vi "AlliGator Image Pre-processing.vi"(5 "Image Pre-Processing Parameters":T1 {"Hot Pixel Removal"."Percentile" min=0 max=100}, 6 "Data":sgl[][](array[numeric]), 7 "Buffer Image available?":bool, 8 "error in (no error)":errorcluster, 9 "Current Gate":i32, 10 "Refnum in":T6, 11 "Dataset Images in":T7) -> (0 "error out":errorcluster, 1 "Current Gate (dup)":i32, 2 "# Replacements":i32, 3 "Dataset Images out":T7, 4 "Image Resolution":cluster{"X Resolution":i32, "Y Resolution":i32})   [LabVIEW 2021, in "AlliGator Files.lvlib"]
doc: "Applies selected preprocessing steps to a gate image."
uses:
  AlliGator Files.lvlib
  AlliGator Gate Image Set.ctl
  <vilib>/vision/Image Controls.llb/IMAQ Image.ctl
  AlliGator Image Pre-processing Parameters.ctl
  Arrays/Kernel Type.ctl
  Arrays/Smoothing Algorithm.ctl
  SwissSPAD/SwissSPAD Live_Image Display Options.ctl
  AlliGator Image Pre-processing Step.ctl
  AlliGator Settings List.ctl
  de9ca15b-1b35-494c-9863-d7c52523ff08.vi
  a9c29a31-92f7-4b3b-9283-b1d6627186df.vi
  Arrays/n x n Kernel Convolution (SGL).vi
  Arrays/n x n Smoothen Array (SGL) v3.vi
  Arrays/n x n Kernel Convolution (SGL).vi/d0ebc029-cbaa-4c82-a58c-923c59c440da.vi
  Arrays/n x n Kernel Convolution (SGL).vi/b80d5e79-a0c8-46e2-aba9-3d60e0093a16.vi
  <vilib>/Analysis/2dsp.llb/Convolution.vi
  <vilib>/Analysis/2dsp.llb/2D Convolution (DBL).vi
  Arrays/Truncate Kernel.vi
  Arrays/Replace NaN by 0 (2D SGL).vi
  Arrays/n x n Smoothen Array (SGL) v3.vi/d0ebc029-cbaa-4c82-a58c-923c59c440da.vi
  Arrays/n x n Smoothen Array (SGL) v3.vi/b80d5e79-a0c8-46e2-aba9-3d60e0093a16.vi
  Arrays/Replace NaN by 0 (2D SGL).vi/df975b44-f6c5-4554-af30-980613d33749.vi
  Variant/Variant to Data/Variant to Boolean.vi
  Time/High Resolution Timing.vi
  Arrays/Compute n x n Kernel (SGL).vi
  <vilib>/Utility/error.llb/Simple Error Handler.vi
  Arrays/Arrays.lvlib
  AlliGator Settings.lvlib
  Variant/Variant to Data/Variant to Data.lvlib
  AlliGator Internal Variables.lvlib
  SwissSPAD/SwissSPAD Live.lvlib
panel:
  # "see the AlliGator License on the block diagram (Ctrl+E or Window:Show Block Diagram)"
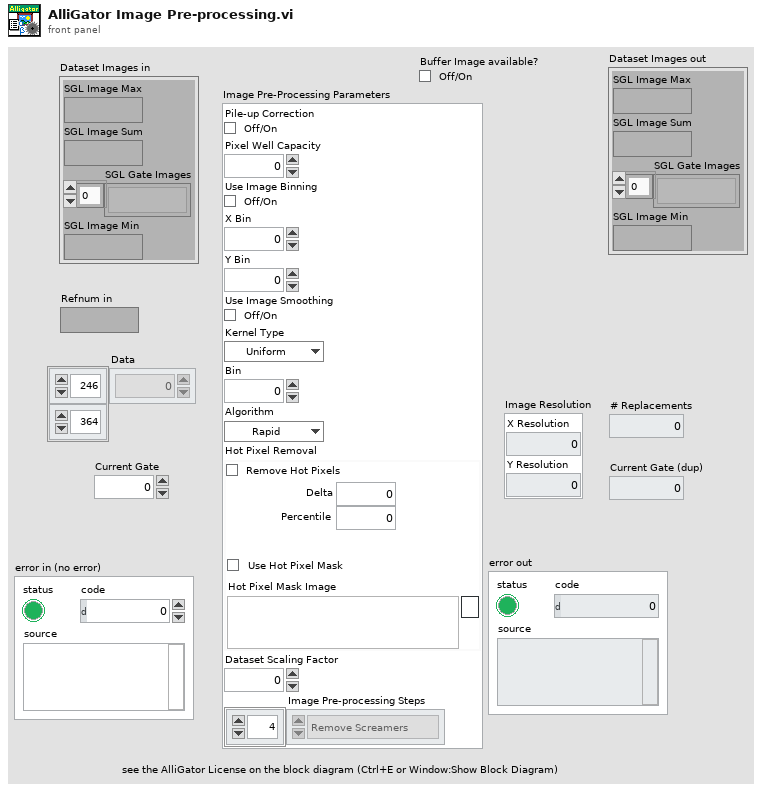
[diagram p1: front panel]
types:
  T1 = typedef "AlliGator Files.lvlib/AlliGator Image Pre-processing Parameters.ctl" = cluster{"Pile-up Correction":bool, "Pixel Well Capacity":u32, "Use Image Binning":bool, "X Bin":i32, "Y Bin":i32, "Use Image Smoothing":bool, "Kernel Type":T2, "Bin":i32, "Algorithm":T3, "Hot Pixel Removal":T4, "Dataset Scaling Factor":dbl, "Image Pre-processing Steps":T5[]}
  T2 = typedef "Arrays.lvlib/Kernel Type.ctl" = enum16{"Uniform", "Bilinear", "Gaussian"}
  T3 = typedef "Arrays.lvlib/Smoothing Algorithm.ctl" = enum16{"Rapid", "Thorough"}
  T4 = typedef "SwissSPAD Live.lvlib/SwissSPAD Live_Image Display Options.ctl" = cluster{"Remove Screamers":bool, "Delta":sgl, "Equalize Histogram":bool, "Percentile":sgl, "Hot Pixel Mask Image":path, "Use Hot Pixel Mask":bool}
  T5 = typedef "AlliGator Files.lvlib/AlliGator Image Pre-processing Step.ctl" = enum16{"Remove Screamers", "Pile-up Correction", "Binning", "Smoothing", "Rescaling", "Dead Left Column Correction"}
  T6 = typedef "IMAQ Image.ctl" = refnum<image>
  T7 = typedef "AlliGator Internal Variables.lvlib/AlliGator Gate Image Set.ctl" = cluster{"SGL Image Max":T6, "SGL Image Sum":T6, "SGL Gate Images":T6[], "SGL Image Min":T6}
  T8 = typedef "AlliGator Settings.lvlib/AlliGator Settings List.ctl" = enum16{"GUI:Visible Settings Tab", "GUI:Last Run Version", "Source Image:Use Image Histogram for Contrast", "Source Image:Low Count Pixels Rejection Options", "Source Image:High Count Pixels Rejection Options", "Source Image:Use Image Brightness", "Source Image:Blend Overlay with Image Background", "Source Image:Use Fixed ROI Diameter", "Source Image:ROI Diameter", "Source Image:ROI Center Color", "Source Image:Peak Threshold", "Source Image:Intensity Threshold", "Source Image:Image Binning Options", "Source Image:Image Smoothing Options", "Source Image:Image Histogram Active", "Source Image:Invert Binary Mask", "Source Image:Hot Pixel Removal", "Source Image:Overlay Analyzed ROI Center", "Source Image:Auto-Adjust Contrast", "Source Image:Histogram Lower Percentile", "Source Image:Histogram Upper Percentile", "Source Image:Save Source Image", "Source Image:Scale Bar Options", "Source Image:Image Resolution (Pixel Size)", "Source Image:Flatfield Correction", "Source Image:Show Dead Left Columns Correction", "Source Image:Dead Left Columns Correction", "Source Image:Image Pre-Processing Operations Order", "Data Information:Gate Width", "Data Information:Nanotime Gate Separation", "Data Information:Macrotime Gate Separation", "Data Information:Gate Step", "Data Information:# Gates", "Data Information:Gate Image Exposure", "Data Information:Gate Image Integration", "Data Information:Gates to Skip", "Data Information:Gates to Keep", "Data Information:Define Gates to", "Data Information:Channel Name", "Data Information:Available Channel Names", "Data Information:Channel Arithmetic", "Data Information:Background File Subtraction", "Data Information:Background File", "Data Information:Background Scaling Factor", "Data Information:Background Pile-up Correction", "Data Information:Background Pixel Well Capacity", "Data Information:Laser Period", "Data Information:SYNC Period", "Data Information:Pile-up Correction", "Data Information:Pixel Well Capacity", "Data Information:Dataset Scaling Factor", "Fluorescence Decay_Decay Pre-Processing:Reverse Gates", "Fluorescence Decay_Decay Pre-Processing:Verbose Decay Pre-Processing", "Fluorescence Decay_Decay Pre-Processing:Use Decay Pre-Processing", "Fluorescence Decay_Decay Pre-Processing:Background Subtraction", "Fluorescence Decay_Decay Pre-Processing:Background Definition Range", "Fluorescence Decay_Decay Pre-Processing:Baseline Subtraction Method", "Fluorescence Decay_Decay Pre-Processing:Decay Pre-Processing Operations Order", "Fluorescence Decay_Decay Pre-Processing:Smoothing Parameter", "Fluorescence Decay_Decay Pre-Processing:Shift Decay", "Fluorescence Decay_Decay Pre-Processing:Decay Shift Parameters", "Fluorescence Decay_Decay Pre-Processing:Fold Decay", "Fluorescence Decay_Decay Pre-Processing:# Folds", "Fluorescence Decay_Decay Pre-Processing:1-Normalize Decay", "Fluorescence Decay_Decay Pre-Processing:[0-1]-Normalize Decay", "Fluorescence Decay_Decay Pre-Processing:Smoothen Decay", "Fluorescence Decay_Decay Pre-Processing:Extrapolate Decay", "Fluorescence Decay_Decay Pre-Processing:Use Periodicity", "Fluorescence Decay_Decay Pre-Processing:Use Cursors", "Fluorescence Decay_Decay Pre-Processing:Tail Fraction", "Fluorescence Decay_Decay Pre-Processing:Head Fraction", "Fluorescence Decay_Decay Pre-Processing:Additional Points", "Fluorescence Decay_Decay Pre-Processing:Straighten Decay", "Fluorescence Decay_Decay Pre-Processing:Constant Background", "Fluorescence Decay_Decay Pre-Processing:Pixel-Normalize Decay", "Fluorescence Decay_Advanced Analysis:Extract IRF instead of Decay", "Fluorescence Decay_Advanced Analysis:IRF Extraction Options", "Fluorescence Decay_Advanced Analysis:IRF Optimization Options", "Fluorescence Decay_Advanced Analysis:Square Pulse Options", "Fluorescence Decay_Advanced Analysis:IRF Order", "Fluorescence Decay_Advanced Analysis:IRF Time Constants", "Fluorescence Decay_Advanced Analysis:Wavelet Analysis Options", "Fluorescence Decay_Advanced Analysis:Average Lifetime Options", "Fluorescence Decay_Fit Options:Fit Options", "Fluorescence Decay_Fit Options:Use Legacy Fitting Approach", "Fluorescence Decay_Fit Options:Use Data Information Laser Period", "Fluorescence Decay_Fit Parameters:Displayed Fit Parameters", "Fluorescence Decay_Fit Parameters:Fit Parameter Constraints", "Fluorescence Decay_Fit Parameters:Export Tabulated Results", "Fluorescence Decay_Fit Parameters:MLE Baseline Offset Type", "Fluorescence Decay_Fit Parameters:MLE Baseline Offset", "Fluorescence Decay_Fit Parameters:Guess Parameter Names", "Fluorescence Decay_Fit Parameters:Guess Parameter Values", "Fluorescence Decay_Fit Parameters:Guess Parameters Options", "Fluorescence Decay_Styles:Show Last Decay Only", "Fluorescence Decay_Styles:Decay Graph Color Array", "Fluorescence Decay:Decay Graph Active", "Fluorescence Decay Statistics:Min Peak Value", "Fluorescence Decay Statistics:Reject Low Decay Peak Pixels", "Fluorescence Decay Statistics:Reject High Decay Peak Pixels", "Fluorescence Decay Statistics:Max Peak Value", "Time Traces:Use File Timestamp", "Time Traces:Time Step", "Time Traces:Use Intensity Correction File", "Time Traces:Intensity Correction File", "Phasor Plot:Phasor Plot Smoothing Options", "Phasor Plot:Phasor Plot Size", "Phasor Plot:Phasor Plot Graphics Options", "Phasor Plot:Cumulative Phasor Plot", "Phasor Plot:Use Phasor Brightness", "Phasor Plot:Blend Overlay with Phasor Background", "Phasor Plot:Save Phasor Plot", "Phasor Plot:Show References", "Phasor Plot:Phasor Ratio Decay Range", "Phasor Plot:Exponential Fading", "Phasor Plot:Phasor Ratio Reference Colors", "Phasor Plot:Reference Radius", "Phasor Plot:Show Color Map Vertices", "Phasor Plot:Phasor Plot Active", "Phasor Plot:Phasor Ratio Color Map Type", "Phasor Plot:Phasor Ratio Color Map", "Phasor Plot:Phasor Ratio Display Range", "Phasor Plot:Selected Image ROI(s)", "Phasor Plot:All Image ROIs", "Phasor Plot:Selected Phasor Plot ROI(s)", "Phasor Plot:All Phasor Plot ROIs", "Phasor Plot:Phasor Ratio Color-Coded Quantity", "Phasor Plot:Store Phasor Harmonics", "Phasor Plot:Draw Reference Segment", "Phasor Plot:User-Defined Quantity", "Phasor Graph:Phasor Frequency", "Phasor Graph:Phasor Ratio Type", "Phasor Graph:Pixel-level Phasor Computation", "Phasor Graph:Save Phasor Graph", "Phasor Graph:Phasor Graph Active", "Phasor Graph:Phasor SDV Options", "Phasor Calibration:Use Backup Calibration if needed", "Phasor Graph:Define Shortest Lifetime as", "Phasor Calibration:Backup Calibration Type", "Phasor Calibration:Calibration Type", "Phasor Calibration:Calibration Lifetime", "Phasor Calibration:Calibration Map Algorithm", "Single-Exponential Phasor Locus (SEPL):Gate Parameters", "Single-Exponential Phasor Locus (SEPL):User-defined Gate", "Single-Exponential Phasor Locus (SEPL):User-defined IRF", "Single-Exponential Phasor Locus (SEPL):Phasor Parameters", "Single-Exponential Phasor Locus (SEPL):Decay & IRF Parameters", "Single-Exponential Phasor Locus (SEPL):Display Parameters", "Lifetime Analysis:Decay Analysis Parameters", "Lifetime Analysis:Lifetime Map Active", "Plugins:Python Settings", "Miscellaneous:Verbose Mode", "Miscellaneous:Beep after Script", "Miscellaneous:Saved Image File Format", "Miscellaneous:Exported Gate Image Settings", "Miscellaneous:Include Loading in Timing", "Miscellaneous:Verbose Settings Mode", "Miscellaneous:Histogram Options", "Miscellaneous:Beep on Error", "Miscellaneous:# Logical Processors Used", "Miscellaneous:ROI Description Max Characters", "Miscellaneous:Verbose Error Mode", "Miscellaneous:Transparent Mask Color"}
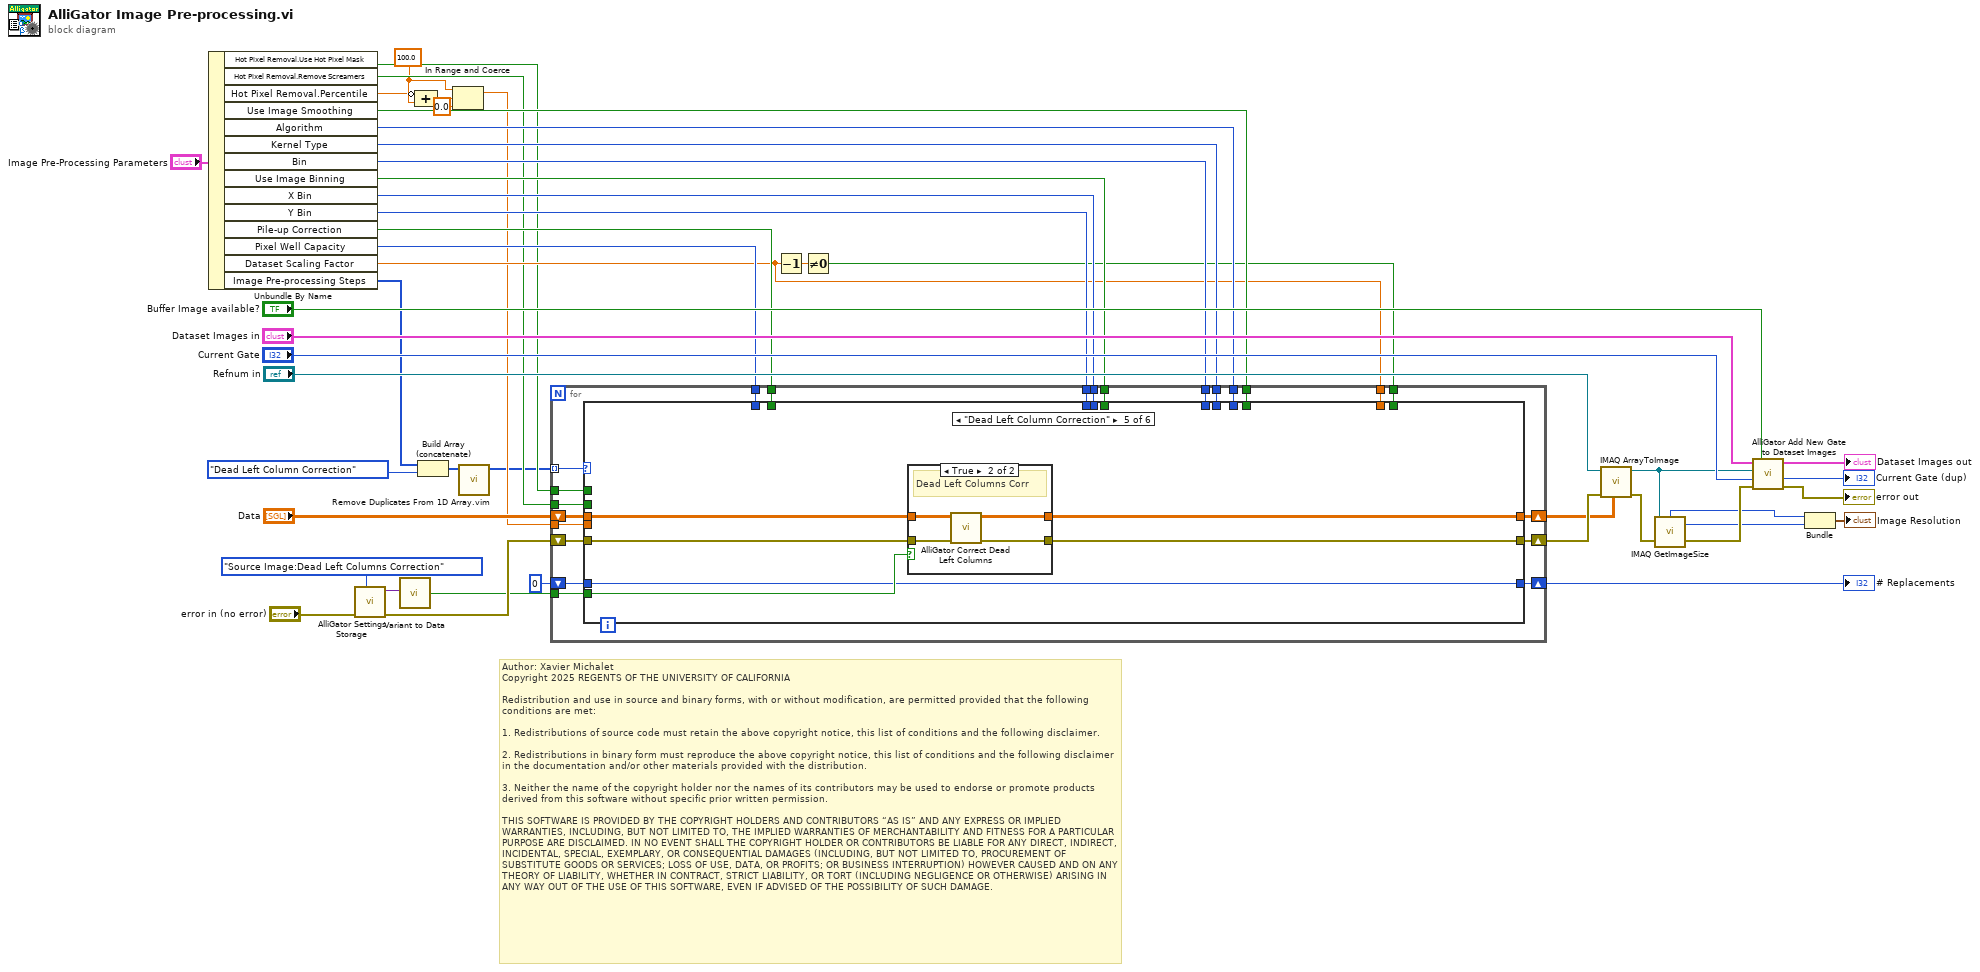
[diagram p0: block diagram]
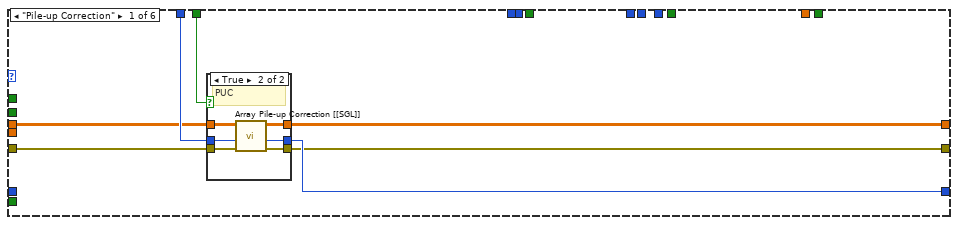
[diagram p2: hidden frame]
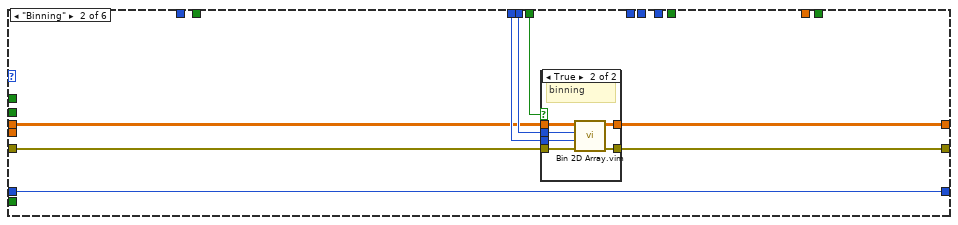
[diagram p4: hidden frame]
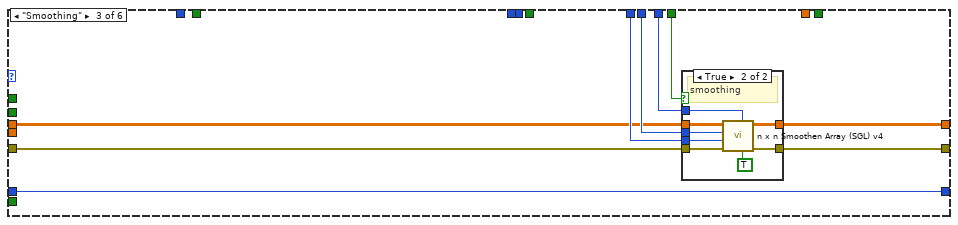
[diagram p6: hidden frame]
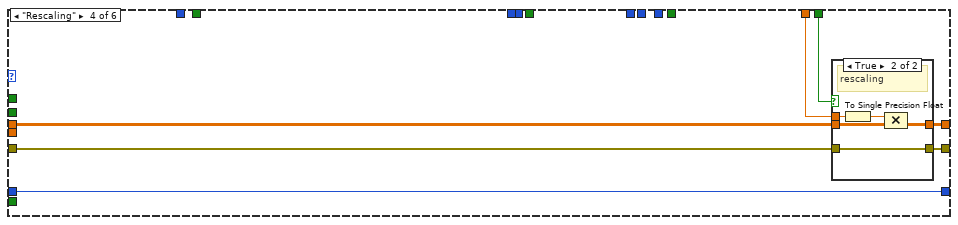
[diagram p8: hidden frame]
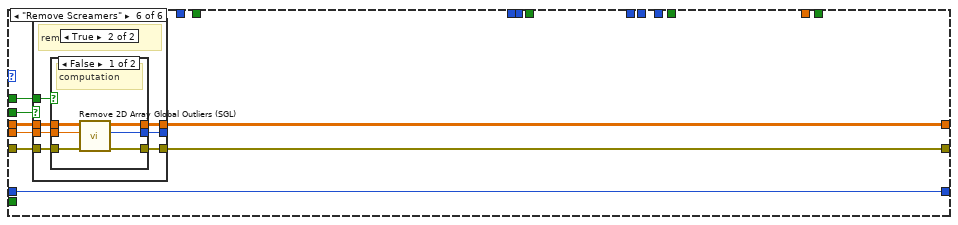
[diagram p11: hidden frame]
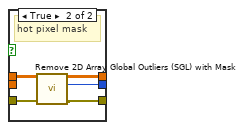
[diagram p13: hidden frame]
diagram:
  w14 = sgl 100.0 ("value")
  # "Author: Xavier Michalet\nCopyright 2025 REGENTS OF THE UNIVERSITY OF CALIFORNIA\n\nRedistribution and use in source and binary forms, with or without modification, are permitted provided that the following conditions are met:\n\n1. Redistributions of source code must retain the above copyright notice, this list of conditions and the following disclaimer.\n\n2. Redistributions in binary form must reproduce the above copyright notice, this list of conditions and the following disclaimer in the documentation and/or other materials provided with the distribution.\n\n3. Neither the name of the copyright holder nor the names of its contributors may be used to endorse or promote products derived from this software without specific prior written permission.\n\nTHIS SOFTWARE IS PROVIDED BY THE COPYRIGHT HOLDERS AND CONTRIBUTORS “AS IS” AND ANY EXPRESS OR IMPLIED WARRANTIES, INCLUDING, BUT NOT LIMITED TO, THE IMPLIED WARRANTIES OF MERCHANTABILITY AND FITNESS FOR A PARTICULAR PURPOSE ARE DISCLAIMED. IN NO EVENT SHALL THE COPYRIGHT HOLDER OR CONTRIBUTORS BE LIABLE FOR ANY DIRECT, INDIRECT, INCIDENTAL, SPECIAL, EXEMPLARY, OR CONSEQUENTIAL DAMAGES (INCLUDING, BUT NOT LIMITED TO, PROCUREMENT OF SUBSTITUTE GOODS OR SERVICES; LOSS OF USE, DATA, OR PROFITS; OR BUSINESS INTERRUPTION) HOWEVER CAUSED AND ON ANY THEORY OF LIABILITY, WHETHER IN CONTRACT, STRICT LIABILITY, OR TORT (INCLUDING NEGLIGENCE OR OTHERWISE) ARISING IN ANY WAY OUT OF THE USE OF THIS SOFTWARE, EVEN IF ADVISED OF THE POSSIBILITY OF SUCH DAMAGE."
  n1 = Unbundle By Name("Image Pre-Processing Parameters") -> ("Hot Pixel Removal.Use Hot Pixel Mask"=w16:bool, "Hot Pixel Removal.Remove Screamers"=w17:bool, "Hot Pixel Removal.Percentile"=w12:sgl, "Use Image Smoothing"=w34:bool, "Algorithm"=w31:T3, "Kernel Type"=w33:T2, "Bin"=w32:i32, "Use Image Binning"=w37:bool, "X Bin"=w36:i32, "Y Bin"=w35:i32, "Pile-up Correction"=w39:bool, "Pixel Well Capacity"=w38:u32, "Dataset Scaling Factor"=w19:dbl, "Image Pre-processing Steps"=w4:T5[])
  n2 = call "AlliGator Settings Storage.vi"("AlliGator Settings List"=AlliGator_Settings_List."Source Image:Dead Left Columns Correction", "Error In"="error in (no error)") -> ("Error Out"=w9:errorcluster, "Variant Data out"=w7:variant)  [unwired: 8 in]
  n3 = call-poly "Variant to Data.vi"("Variant"=w7) -> ("Value"=w6:bool)  [unwired: 8 in]
  n4 = Compound Arithmetic op=ADD(invert w12, w14) -> (w13:sgl)
  n5 = Build Array (concatenate)(w4, AlliGator_Image_Pre-processing_Step."Dead Left Column Correction" ("array")) -> (w3:T5[])
  n6 = In Range and Coerce(upper limit=w14, x=w13, lower limit=sgl 0.0) -> (coerced(x)=w11:sgl)  [unwired: 1 out]
  n7 = call "Remove Duplicates From 1D Array.vim"("array"=w3) -> ("array with duplicates removed"=w1:T5[])  [unwired: 10 in]
  n8 = Decrement(x=w19) -> (x-1=w23:dbl)
  n9 = Not Equal To 0?(x=w23) -> (x != 0?=w22:bool)
  n10 = for {
    tunnel: w39 -> [w68]
    tunnel: w38 -> [w67]
    tunnel: w37 -> [w66]
    tunnel: w36 -> [w65]
    tunnel: w35 -> [w64]
    tunnel: w34 -> [w63]
    tunnel: w33 -> [w62]
    tunnel: w32 -> [w61]
    tunnel: w31 -> [w60]
    tunnel: w22 -> [w59]
    tunnel: w19 -> [w56]
    tunnel: w17 -> [w54]
    tunnel: w16 -> [w53]
    tunnel: w11 -> [w52]
    tunnel: w6 -> [w50]
    shift-right: [w58] -> w21
    shift-left: w9 -> [w51]
    shift-right: [w57] -> w20
    shift-left: "Data" -> [w55]
    tunnel: w1 -> [w49] mode=indexing
    shift-right: [w69] -> w41
    shift-left: 0 ("# Replacements") -> [w48]
    n11 = case shown="\"Dead Left Column Correction\"" w49 {
      tunnel: [w76 w85 w101 w120 w134 w146] -> w69
      tunnel: w68 -> [w73 _ _ _ _ _]
      tunnel: w67 -> [w72 _ _ _ _ _]
      tunnel: w66 -> [_ w90 _ _ _ _]
      tunnel: w65 -> [_ w89 _ _ _ _]
      tunnel: w64 -> [_ w88 _ _ _ _]
      tunnel: w63 -> [_ _ w109 _ _ _]
      tunnel: w62 -> [_ _ w108 _ _ _]
      tunnel: w61 -> [_ _ w107 _ _ _]
      tunnel: w60 -> [_ _ w106 _ _ _]
      tunnel: w59 -> [_ _ _ w126 _ _]
      tunnel: [w74 w91 w104 w125 w137 w149] -> w58
      tunnel: [w75 w92 w105 w124 w136 w150] -> w57
      tunnel: w56 -> [_ _ _ w123 _ _]
      tunnel: w55 -> [w71 w87 w103 w122 w139 w153]
      tunnel: w54 -> [_ _ _ _ _ w152]
      tunnel: w53 -> [_ _ _ _ _ w151]
      tunnel: w52 -> [_ _ _ _ _ w148]
      tunnel: w51 -> [w70 w86 w102 w121 w138 w147]
      tunnel: w50 -> [_ _ _ _ w135 _]
      tunnel: w48 -> [_ w85 w101 w120 w134 w146]
      frame "Pile-up Correction" {
        n12 = case shown="True" w73 {
          tunnel: w71 -> [w77 w80]
          tunnel: w70 -> [w78 w84]
          tunnel: w72 -> [_ w83]
          tunnel: [w78 w82] -> w74
          tunnel: [w77 w79] -> w75
          tunnel: [_ w81] -> w76
          frame False {
            # "no PUC"
          }
          frame True {
            # "PUC"
            n13 = call "Array Pile-up Correction [[SGL]].vi"("Error In"=w84, "Pixel well capacity"=w83, "Image Pixels"=w80) -> ("Error Out"=w82:errorcluster, "# Replacements"=w81:i32, "Corrected Image Pixels"=w79:sgl[][])  [unwired: 6 in]
          }
        }
      }
      frame "Binning" {
        n14 = case shown="True" w90 {
          tunnel: w86 -> [w93 w100]
          tunnel: [w93 w99] -> w91
          tunnel: w89 -> [_ w98]
          tunnel: w88 -> [_ w97]
          tunnel: w87 -> [w94 w96]
          tunnel: [w94 w95] -> w92
          frame False {
            # "no binning"
          }
          frame True {
            # "binning"
            n15 = call "Bin 2D Array.vim"("Error In"=w100, "Y Bin (1)"=w97, "X Bin (1)"=w98, "Array"=w96) -> ("Error Out"=w99:errorcluster, "Binned Array"=w95:sgl[][])  [unwired: 2 in, 4 out]
          }
        }
      }
      frame "Smoothing" {
        n16 = case shown="True" w109 {
          tunnel: w102 -> [w110 w119]
          tunnel: [w110 w118] -> w104
          tunnel: [w111 w117] -> w105
          tunnel: w103 -> [w111 w116]
          tunnel: w108 -> [_ w115]
          tunnel: w107 -> [_ w114]
          tunnel: w106 -> [_ w112]
          frame False {
            # "no smoothing"
          }
          frame True {
            # "smoothing"
            n17 = call "n x n Smoothen Array (SGL) v4.vi"("Average"=TRUE, "Algorithm"=w112, "Error In"=w119, "Kernel Size"=w114, "Kernel Type"=w115, "Array in"=w116) -> ("Error Out"=w118:errorcluster, "Array out"=w117:sgl[][])  [unwired: 3 in, 1 out]
          }
        }
      }
      frame "Rescaling" {
        n18 = case shown="True" w126 {
          tunnel: w122 -> [w127 w133]
          tunnel: w121 -> [w128 w130]
          tunnel: [w128 w130] -> w125
          tunnel: [w127 w131] -> w124
          tunnel: w123 -> [_ w132]
          frame False {
            # "no scaling"
          }
          frame True {
            # "rescaling"
            n19 = To Single Precision Float(number=w132) -> (single precision float=w129:sgl)
            n20 = Compound Arithmetic op=MULTIPLY(w129, w133) -> (w131:sgl[][])
          }
        }
      }
      frame "Dead Left Column Correction" {
        n21 = case shown="True" w135 {
          tunnel: w139 -> [w141 w145]
          tunnel: w138 -> [w140 w144]
          tunnel: [w140 w143] -> w137
          tunnel: [w141 w142] -> w136
          frame False {
          }
          frame True {
            # "Dead Left Columns Corr"
            n22 = call "AlliGator Correct Dead Left Columns.vi"("error in (no error)"=w144, "Image Pixels"=w145) -> ("error out"=w143:errorcluster, "Corrected Image Pixels"=w142:sgl[][])  [unwired: 8 in]
          }
        }
      }
      frame "Remove Screamers" {
        n23 = case shown="True" w152 {
          tunnel: w153 -> [w155 w162]
          tunnel: [w155 w161] -> w150
          tunnel: w147 -> [w154 w160]
          tunnel: [w154 w159] -> w149
          tunnel: w148 -> [_ w158]
          tunnel: [_ w157] -> _
          tunnel: w151 -> [_ w156]
          frame False {
            # "no screamers"
          }
          frame True {
            # "remove screamers"
            n24 = case shown="False" w156 {
              tunnel: w162 -> [w168 w171]
              tunnel: [w167 w170] -> w161
              tunnel: w160 -> [w166 w173]
              tunnel: [w165 w172] -> w159
              tunnel: w158 -> [w164 _]
              tunnel: [w163 w169] -> w157
              frame False {
                # "computation"
                n25 = call "Remove 2D Array Global Outliers (SGL).vi"("Error In"=w166, "Percentile (0-100, Default: ignore)"=w164, "2D Array in"=w168) -> ("Error Out"=w165:errorcluster, "# Modified Values"=w163:i32, "2D Array out"=w167:sgl[][])  [unwired: 6 in]
              }
              frame True {
                # "hot pixel mask"
                n26 = call "Remove 2D Array Global Outliers (SGL) with Mask.vi"("Error In"=w173, "2D Array in"=w171) -> ("Error Out"=w172:errorcluster, "# Modified Values"=w169:i32, "2D Array out"=w170:sgl[][])  [unwired: 7 in]
              }
            }
          }
        }
      }
    }
  }
  "# Replacements" <- w41
  n27 = call "IMAQ ArrayToImage"("Image Pixels (Float)"=w20, "error in (no error)"=w21, "Image"="Refnum in") -> ("error out"=w28:errorcluster, "Image Out"=w29:T6)  [unwired: 7 in]
  n28 = call "IMAQ GetImageSize"("Image"=w29, "error in (no error)"=w28) -> ("Y Resolution"=w25:i32, "X Resolution"=w26:i32, "error out"=w27:errorcluster)  [unwired: 2 in]
  n29 = call "AlliGator Add New Gate to Dataset Images.vi"("Buffer Image available?"="Buffer Image available?", "error in (no error)"=w27, "Current Gate"="Current Gate", "New Gate Image Refnum"=w29, "Dataset Images in"="Dataset Images in") -> ("error out"=→"error out":errorcluster, "Current Gate (dup)"=→"Current Gate (dup)":i32, "Dataset Images out"=→"Dataset Images out":T7)  [unwired: 4 in]
  n30 = Bundle("X Resolution"=w26, "Y Resolution"=w25) -> (→"Image Resolution":cluster{"X Resolution":i32, "Y Resolution":i32})  [unwired: 1 in]
